vi "LVJSON Create Root Path.vi"(8 "error in (no error)":errorcluster, 10 "Element in":T1, 11 "Root Path":string[](array[string])) -> (0 "error out":errorcluster, 3 "Root Element out":T1)   [LabVIEW 2019, in "labview_json.lvlib"]
uses:
  labview_json.lvlib
  Element.ctl
  Element Type.ctl
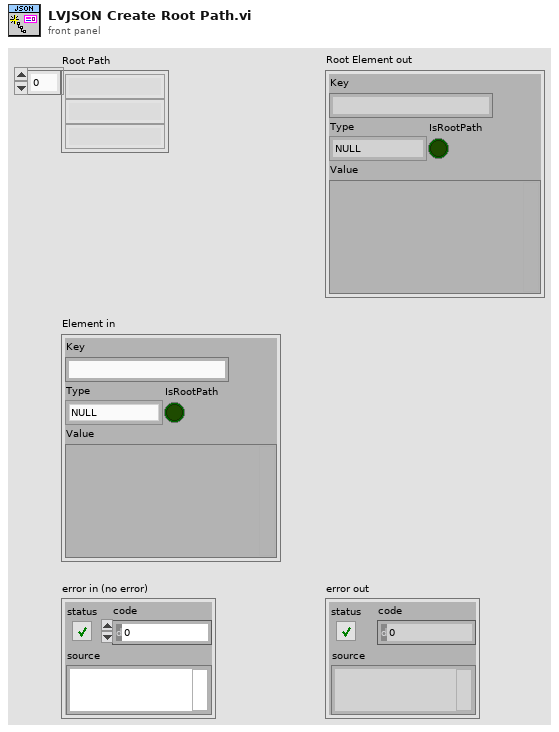
[diagram p1: front panel]
types:
  T1 = typedef "labview_json.lvlib/Element.ctl" = cluster{"Key":string, "Type":T2, "Value":variant, "IsRootPath":bool}
  T2 = typedef "labview_json.lvlib/Element Type.ctl" = enum8{"NULL", "OBJECT", "ARRAY", "BOOL", "INT", "UINT", "FLOAT", "STRING"}
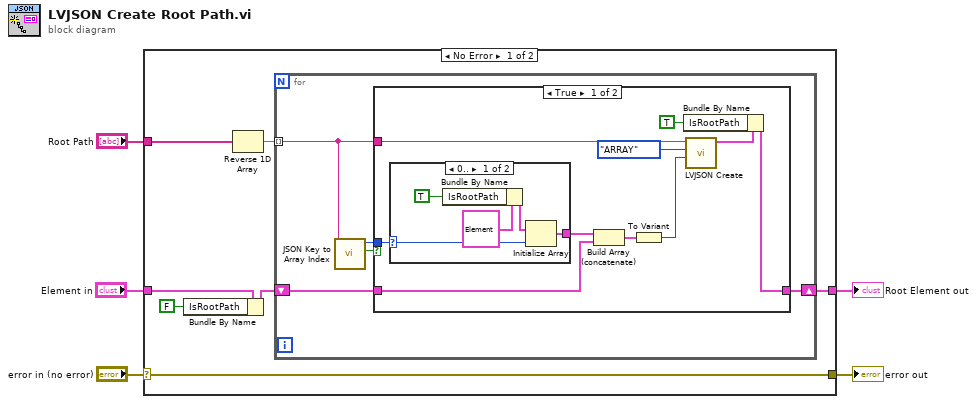
[diagram p0: block diagram]
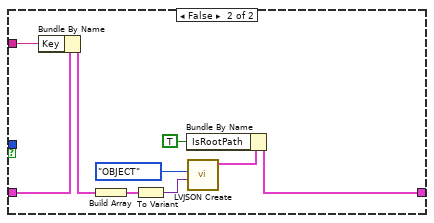
[diagram p3: hidden frame]
diagram:
  n1 = case shown="No Error" "error in (no error)" {
    selector: "error in (no error)" -> [w12 w43]
    tunnel: [w9 w42] -> w5
    tunnel: "Element in" -> [w10 w42]
    tunnel: "Root Path" -> [w11 _]
    tunnel: [w12 w43] -> w2
    frame No Error {
      n2 = Bundle By Name(cluster=w10, "IsRootPath"=FALSE) -> (w7:T1)
      n3 = Reverse 1D Array(array=w11) -> (reversed array=w8:string[])
      n4 = for {
        tunnel: w8 -> [w13] mode=indexing
        shift-right: [w16] -> w9
        shift-left: w7 -> [w17]
        n5 = call "JSON Key to Array Index.vi"("Key"=w13) -> ("Is Index?"=w14:bool, "Index"=w15:i32)  [unwired: 8 in, 1 out]
        n6 = case shown="True" w14 {
          tunnel: w17 -> [w22 w40]
          tunnel: [w19 w34] -> w16
          tunnel: w13 -> [w20 w35]
          tunnel: w15 -> [w24 _]
          frame True {
            n7 = case shown="0.." w24 {
              selector: w24 -> [w32 _]
              tunnel: [w30 _] -> w23
              frame 0.. {
                n8 = Bundle By Name(cluster=T1 {"Key"="", "Type"=enum."NULL", "Value"=variant, "IsRootPath"=FALSE} ("Element out"), "IsRootPath"=TRUE) -> (w29:T1)
                n9 = Initialize Array(w29, w32) -> (w30:T1[])
              }
              frame ..-1 {
              }
            }
            n10 = Build Array (concatenate)(w23, w22) -> (w21:T1[])
            n11 = To Variant(anything=w21) -> (Variant=w27:variant)
            n12 = call "LVJSON Create.vi"("Variant (Void=Default Type)"=w27, "Type"=Element_Type."ARRAY", "Key"=w20) -> ("Element out"=w25:T1)  [unwired: 8 in]
            n13 = Bundle By Name(cluster=w25, "IsRootPath"=TRUE) -> (w19:T1)
          }
          frame False {
            n14 = Bundle By Name(cluster=w40, "Key"=w35) -> (w36:T1)
            n15 = Build Array(w36) -> (w37:T1[])
            n16 = To Variant(anything=w37) -> (Variant=w39:variant)
            n17 = call "LVJSON Create.vi"("Variant (Void=Default Type)"=w39, "Type"=Element_Type."OBJECT") -> ("Element out"=w41:T1)  [unwired: 9 in]
            n18 = Bundle By Name(cluster=w41, "IsRootPath"=TRUE) -> (w34:T1)
          }
        }
      }
    }
    frame Error {
    }
  }
  "error out" <- w2
  "Root Element out" <- w5
